vi "LogAdd (SubVI).vi"(8 "error in":errorcluster, 10 "string":string, 11 "Log":refnum<vi>) -> (0 "error out":errorcluster)   [LabVIEW 2017]
uses:
  Global_SNK3_HF.vi
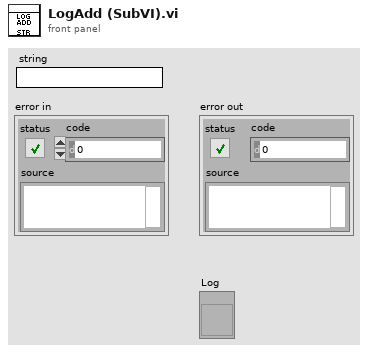
[diagram p1: front panel]
types:
  T1 = enum16{"open", "replace", "create", "open or create", "replace or create", "replace or create with confirmation"}
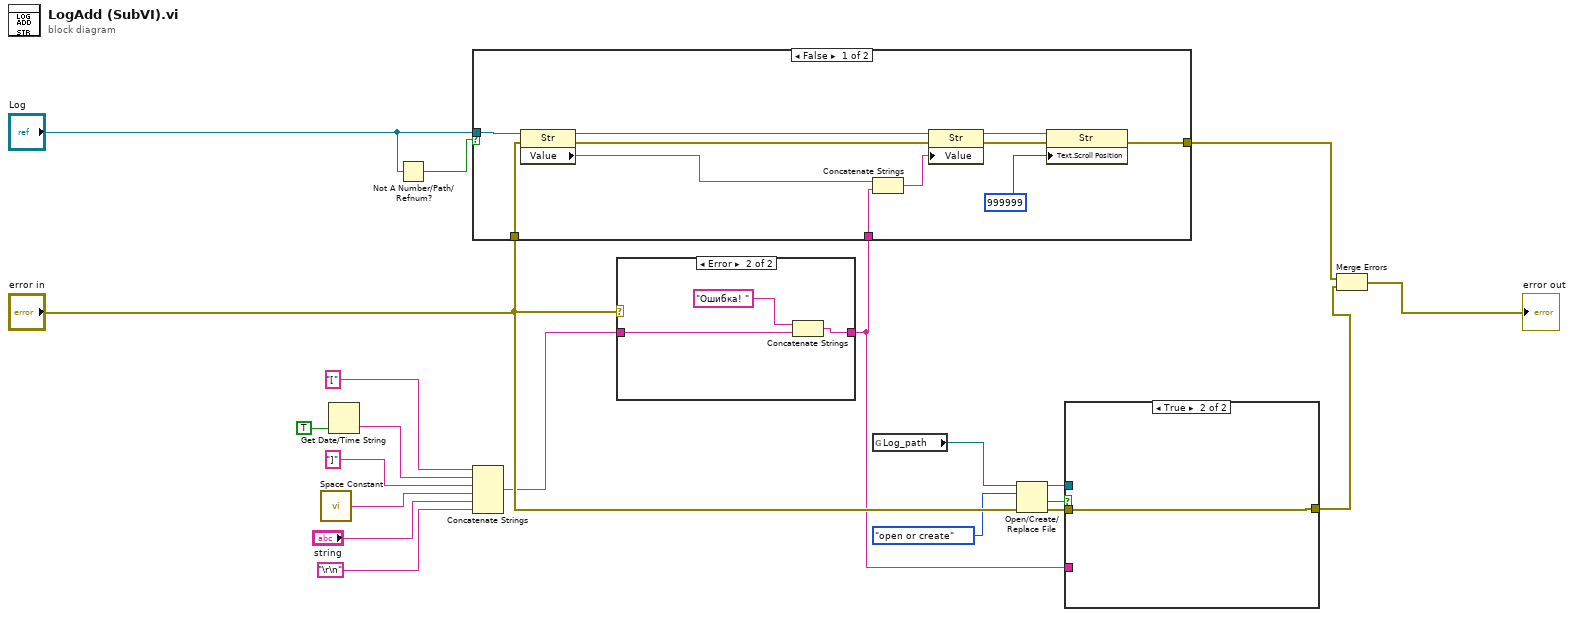
[diagram p0: block diagram]
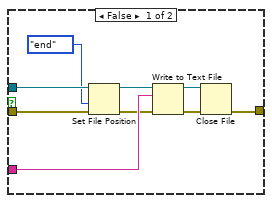
[diagram p3: hidden frame]
diagram:
  n1 = call <vilib>:"Space Constant.vi"() -> ("String"=w16:string)
  n2 = Get Date/Time String(want seconds? (F)=TRUE) -> (time string=w17:string)  [unwired: 2 in, 1 out]
  n3 = Not A Number/Path/Refnum?(number/path/refnum="Log") -> (NaN/Path/Refnum?=w1:bool)
  n4 = Concatenate Strings("[" ("string"), w17, "]" ("string"), w16, "string", "\r\n") -> (w10:string)
  n5 = case shown="Error" "error in" {
    tunnel: w10 -> [w21 w23]
    tunnel: [w21 w22] -> w9
    frame No Error {
    }
    frame Error {
      n6 = Concatenate Strings("Ошибка! " ("string"), w23) -> (w22:string)
    }
  }
  n7 = case shown="False" w1 {
    tunnel: "Log" -> [w28 _]
    tunnel: w9 -> [w27 _]
    tunnel: "error in" -> [w26 w36]
    tunnel: [w25 w36] -> w2
    frame False {
      n8 = property class="Str"(reference=w28, error in=w26) -> (reference out=w35:refnum<vi>, error out=w34:errorcluster, "Value"=w33:string)
      n9 = Concatenate Strings(w33, w27) -> (w32:string)
      n10 = property class="Str"(reference=w35, error in=w34, "Value"=w32) -> (reference out=w31:refnum<vi>, error out=w30:errorcluster)
      n11 = property on="Property Node" class="Str"(reference=w31, error in=w30, "Text.Scroll Position"=u32 999999) -> (error out=w25:errorcluster)  [unwired: 1 out]
    }
    frame True {
    }
  }
  n12 = global read "Global_SNK3_HF.vi" "Log_path"() -> (w7:path)
  n13 = Open/Create/Replace File(file path (use dialog)=w7, error in="error in", operation (0:open)=T1."open or create") -> (refnum out=w4:refnum<file>, cancelled=w5:bool, error out=w6:errorcluster)  [unwired: 3 in]
  n14 = case shown="True" w5 {
    tunnel: w9 -> [w45 _]
    tunnel: w6 -> [w41 w46]
    tunnel: w4 -> [w38 _]
    tunnel: [w42 w46] -> w3
    frame False {
      n15 = Set File Position(refnum=w38, from (0:start)=enum16{"start", "end", "current"}."end", error in=w41) -> (refnum out=w39:refnum<file>, error out=w40:errorcluster)  [unwired: 1 in]
      n16 = Write to Text File(file (use dialog)=w39, text=w45, error in=w40) -> (refnum out=w43:refnum<file>, error out=w44:errorcluster)  [unwired: 1 in, 1 out]
      n17 = Close File(refnum=w43, error in=w44) -> (error out=w42:errorcluster)  [unwired: 1 out]
    }
    frame True {
    }
  }
  n18 = Merge Errors(w2, w3) -> (→"error out":errorcluster)
